vi "KE622x -- Set Arm Timer Interval.vi"(0 "Resource In":refnum<visa-resource-name>, 1 "Check For SCPI Errors? (T)":bool=TRUE, 7 "Arm Timer Interval (s)":T1=0.001 min=0.001 max=99999.999 step=0.001 format="%.3f", 11 "error in (no error)":errorcluster, 12 "Read Back Set Value? (T)":bool=TRUE) -> (4 "Resource Out (dupl)":refnum<visa-resource-name>, 8 "Arm Timer Interval Out (s)":T1 min=0.0 max=99999.999 step=0.001 format="%.3f", 15 "error out":errorcluster)   [LabVIEW 2018, in "Keithley 622x.lvlib"]
uses:
  Keithley 622x.lvlib
  Typedefs/KE622x -- Arm Timer Interval.ctl
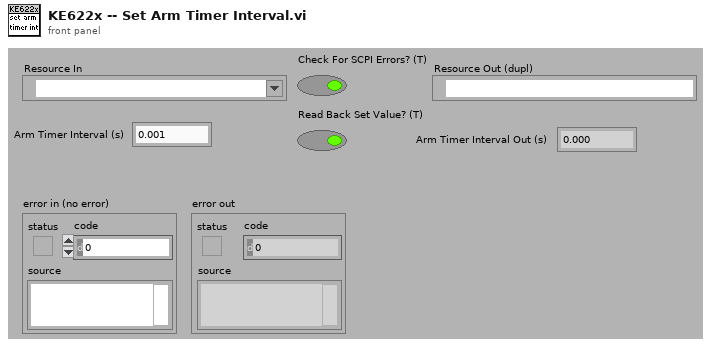
[diagram p1: front panel]
types:
  T1 = typedef "Keithley 622x.lvlib/KE622x -- Arm Timer Interval.ctl" = dbl
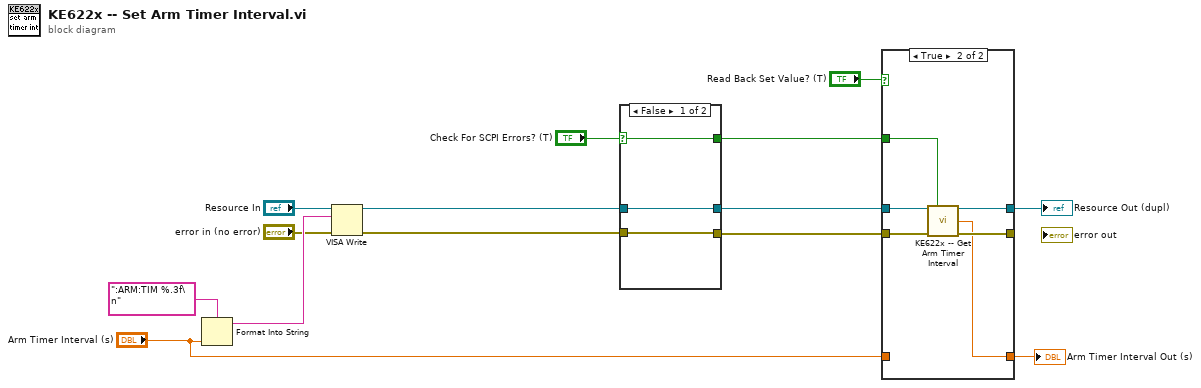
[diagram p0: block diagram]
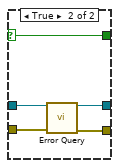
[diagram p3: hidden frame]
diagram:
  n1 = Format Into String(format string=":ARM:TIM %.3f\n", "Arm Timer Interval (s)") -> (resulting string=w12:string)  [unwired: 2 in, 1 out]
  n2 = VISA Write(VISA resource name="Resource In", write buffer=w12, error in (no error)="error in (no error)") -> (VISA resource name out=w9:refnum<visa-resource-name>, error out=w8:errorcluster)  [unwired: 1 out]
  n3 = case shown="False" "Check For SCPI Errors? (T)" {
    selector: "Check For SCPI Errors? (T)" -> [w15 w18]
    tunnel: w9 -> [w17 w22]
    tunnel: w8 -> [w16 w21]
    tunnel: [w16 w20] -> w4
    tunnel: [w17 w19] -> w6
    tunnel: [w15 w18] -> w5
    frame False {
    }
    frame True {
      n4 = call "Error Query.vi"("VISA Resource In"=w22, "error in (no error)"=w21) -> ("VISA Resource Out (dupl)"=w19:refnum<visa-resource-name>, "error out"=w20:errorcluster)  [unwired: 10 in, 2 out]
    }
  }
  n5 = case shown="True" "Read Back Set Value? (T)" {
    tunnel: w6 -> [w24 w31]
    tunnel: w5 -> [_ w30]
    tunnel: w4 -> [w23 w29]
    tunnel: "Arm Timer Interval (s)" -> [w25 _]
    tunnel: [w25 w26] -> w3
    tunnel: [w24 w28] -> w2
    tunnel: [w23 w27] -> _
    frame False {
    }
    frame True {
      n6 = call "KE622x -- Get Arm Timer Interval.vi"("Resource In"=w31, "Check For SCPI Errors? (T)"=w30, "error in (no error)"=w29) -> ("Resource Out (dupl)"=w28:refnum<visa-resource-name>, "Arm Timer Interval (s)"=w26:T1, "error out"=w27:errorcluster)  [unwired: 10 in]
    }
  }
  "Resource Out (dupl)" <- w2
  "Arm Timer Interval Out (s)" <- w3
